vi "Idle.vi"(8 "error in (no error)":errorcluster, 11 "BaseDriver in":refnum<class "BaseDriver.lvclass">) -> (0 "error out":errorcluster, 3 "BaseDriver out":refnum<class "BaseDriver.lvclass">)   [LabVIEW 2013, in "BaseDriver.lvclass"]
doc: "When no data to send or read to/from the remote destination, waits for any to become available"
uses:
  BaseDriver.lvclass
  BaseDriver.lvclass/BaseDriver.ctl
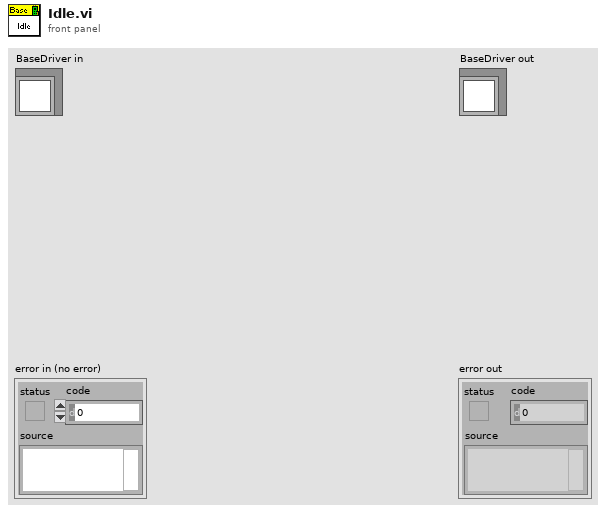
[diagram p1: front panel]
types:
  T1 = typedef "message_queue.ctl" = refnum<queue>
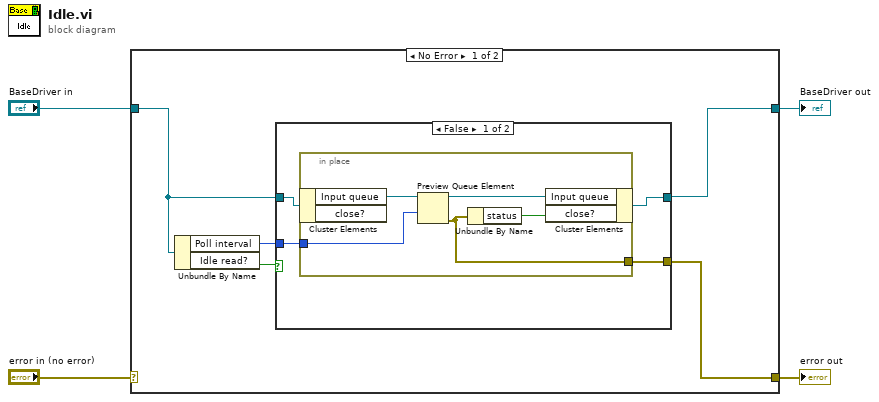
[diagram p0: block diagram]
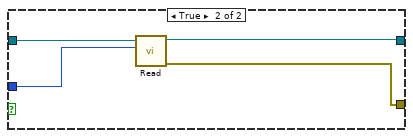
[diagram p2: hidden frame]
diagram:
  n1 = case shown="No Error" "error in (no error)" {
    selector: "error in (no error)" -> [_ w24]
    tunnel: [w5 w24] -> w3
    tunnel: [w6 w23] -> w1
    tunnel: "BaseDriver in" -> [w7 w23]
    frame No Error {
      n2 = Unbundle By Name(w7) -> ("Poll interval"=w8:i32, "Idle read?"=w9:bool)
      n3 = case shown="False" w9 {
        tunnel: w7 -> [w10 w22]
        tunnel: w8 -> [w13 w21]
        tunnel: [w12 w20] -> w6
        tunnel: [w11 w19] -> w5
        frame False {
          n4 = in-place "In Place Element Structure" {
            in-place-border: w13 -> [w16]
            in-place-border: [w15] -> w11
            n5 = in-place-cluster #1(w10) -> ("Input queue"=w18:T1)  [unwired: 1 out]
            n6 = Preview Queue Element(queue=w18, timeout in ms (-1)=w16) -> (queue out=w17:T1, error out=w15:errorcluster)  [unwired: 1 in, 2 out]
            n7 = Unbundle By Name(w15) -> ("status"=w14:bool)
            n8 = in-place-cluster #1("Input queue"=w17, "close?"=w14) -> (w12:refnum<class "BaseDriver.lvclass">)
          }
        }
        frame True {
          n9 = call "Read.vi"("Timeout"=w21, "BaseDriver in"=w22) -> ("error out"=w19:errorcluster, "BaseDriver out"=w20:refnum<class "BaseDriver.lvclass">)  [unwired: 8 in]
        }
      }
    }
    frame Error {
    }
  }
  "error out" <- w3
  "BaseDriver out" <- w1
